vi "globals.vi"() -> ()   [LabVIEW 2010]
panel:
  in  "max bytes":i32=134217728
  # "The maximum number of bytes that a message can be.\n\n\"TCP read.vi\" will stop reading bytes once the message contains the \\r\\n byte sequence.\n\nSet the value as large as you need it to be without running out of memory on your Operating System.\n\nIf you change the value remember to:\nright-click > Data Operations > Make Current Value Default\nand Save the vi.\n\n2**27=134217728=134MB/message"
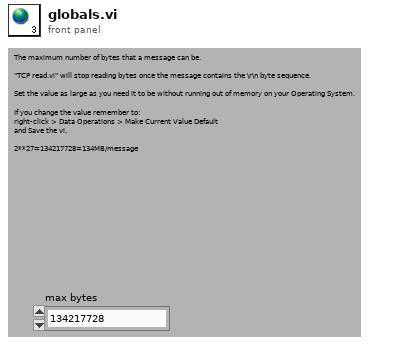
[diagram p1: front panel]
diagram:
